vi "Test WebSocket Upgrade.vi"() -> ()   [LabVIEW 2020]
uses:
  HTTP Server/Trace Log.ctl
  HTTP Server/Trace Item.ctl
  HTTP Server/Processing Step.ctl
  <vilib>/IlluminatedG/IG HTTP Utils/HTTP Utils/Method.ctl
  Test WebSocket Page Controller/Test WebSocket Page Controller.lvclass
  C:/dev/illuminated-g/lv-http-server/HTTP Server/Handler/Handler.lvclass
  <vilib>/IlluminatedG/lv-msg-simple/Stream-Simple-Msg/Format.ctl
  <vilib>/IlluminatedG/lv-stream/stream/Stream.lvclass/Stream.ctl
  ddb143f1-6f1e-4d94-bb27-81deb445b84a.vi
  ddb143f1-6f1e-4d94-bb27-81deb445b84a.vi/2114ae84-1210-427f-82ef-c9e9e7f82752.vi
  <vilib>/IlluminatedG/lv-msg-simple/Stream-Simple-Msg/Endpoint/Write Flattened Data.vi
  ddb143f1-6f1e-4d94-bb27-81deb445b84a.vi/2114ae84-1210-427f-82ef-c9e9e7f82752.vi/850aaa44-16cf-4b05-95d8-204edf60ad4b.vi
  <vilib>/IlluminatedG/lv-stream/stream/Write Data.vi
  ddb143f1-6f1e-4d94-bb27-81deb445b84a.vi/2114ae84-1210-427f-82ef-c9e9e7f82752.vi/850aaa44-16cf-4b05-95d8-204edf60ad4b.vi/c20c7362-1c17-4c7a-86c1-0a7c7649dad4.vi
  <vilib>/IlluminatedG/lv-stream/stream/Dispatch Sniffer Data.vi
  <vilib>/IlluminatedG/lv-stream/stream/Prepared.vi
  <vilib>/IlluminatedG/lv-stream/Endpoint/Cast Sniffer Callback.vi
  <vilib>/IlluminatedG/IG WebSocket Stream/Stream-Websocket/Websocket Server/Websocket Server.lvclass
  C:/Program Files (x86)/National Instruments/LabVIEW 2020/vi.lib/IlluminatedG/lv-stream/Endpoint/Endpoint.lvclass
  HTTP Server/Server/Add Connection Handler.vi
  HTTP Server/Server/Add Request Handler.vi
  HTTP Server/Server/Add Route Handler.vi
  HTTP Server/Server/Add Controller Handler.vi
  HTTP Server/Server/Add Controller.vi
  HTTP Server/Server/Add Response Handler.vi
  HTTP Server/Server/Add Complete Handler.vi
  HTTP Server/Server/Add Exception Handler.vi
  <vilib>/IlluminatedG/lv-msg-simple/Stream-Simple-Msg/Manager/Endpoints and Formats.vi
  <vilib>/IlluminatedG/lv-msg-simple/Stream-Simple-Msg/Endpoint/Get Format.vi
  <vilib>/IlluminatedG/lv-msg-simple/Stream-Simple-Msg/Endpoint/Get Stream.vi
  <vilib>/Utility/error.llb/Error Cluster From Error Code.vi
  HTTP Server/Connection Handler/Connection Handler.lvclass
  HTTP Server/Request Handler/Request Handler.lvclass
  HTTP Server/Route Handler/Route Handler.lvclass
  HTTP Server/Controller Handler/Controller Handler.lvclass
  HTTP Server/Controller/Controller.lvclass
  HTTP Server/Response Handler/Response Handler.lvclass
  HTTP Server/Complete Handler/Complete Handler.lvclass
  HTTP Server/Exception Handler/Exception Handler.lvclass
  <vilib>/IlluminatedG/lv-msg-simple/Stream-Simple-Msg/Manager/Manager.lvclass
  HTTP Server/Server/Server.lvclass
  HTTP Server/Handler/Handler.lvclass
  <vilib>/IlluminatedG/lv-stream/stream/Stream.lvclass
  HTTP Server/RequestTraceLog/RequestTraceLog.lvclass
  <vilib>/ptbypt/NI_PtbyPt.lvlib
  <vilib>/IlluminatedG/lv-msg-simple/Stream-Simple-Msg/Stream-Simple-Msg.lvlib
  WebSocket Test UI Refs/WebSocket Test UI Refs.lvclass
  HTTP Server/HTTP Server.lvlib
  <vilib>/IlluminatedG/IG HTTP Utils/HTTP Utils/HTTP Utils.lvlib
panel:
  out "Last Greeting":string
  out ">0 Clients?":bool
  out "Sine Value":dbl format="%0.2f"
  in  "Refresh Traces":bool
  out "Traces":T1[](array[typedef]) {"Sending" format="%_6f"; "Expires" format="%<%X %x>T"; "Created" format="%<%X %x>T"; "Waiting" format="%_6f"; "Parsing" format="%_6f"; "Processing" format="%_6f"; "Items"."Time" format="%.6f"; "Items"."Duration" format="%.6f"}
  # "Request"
  # "Response"
  # "Session"
  # "Auth"
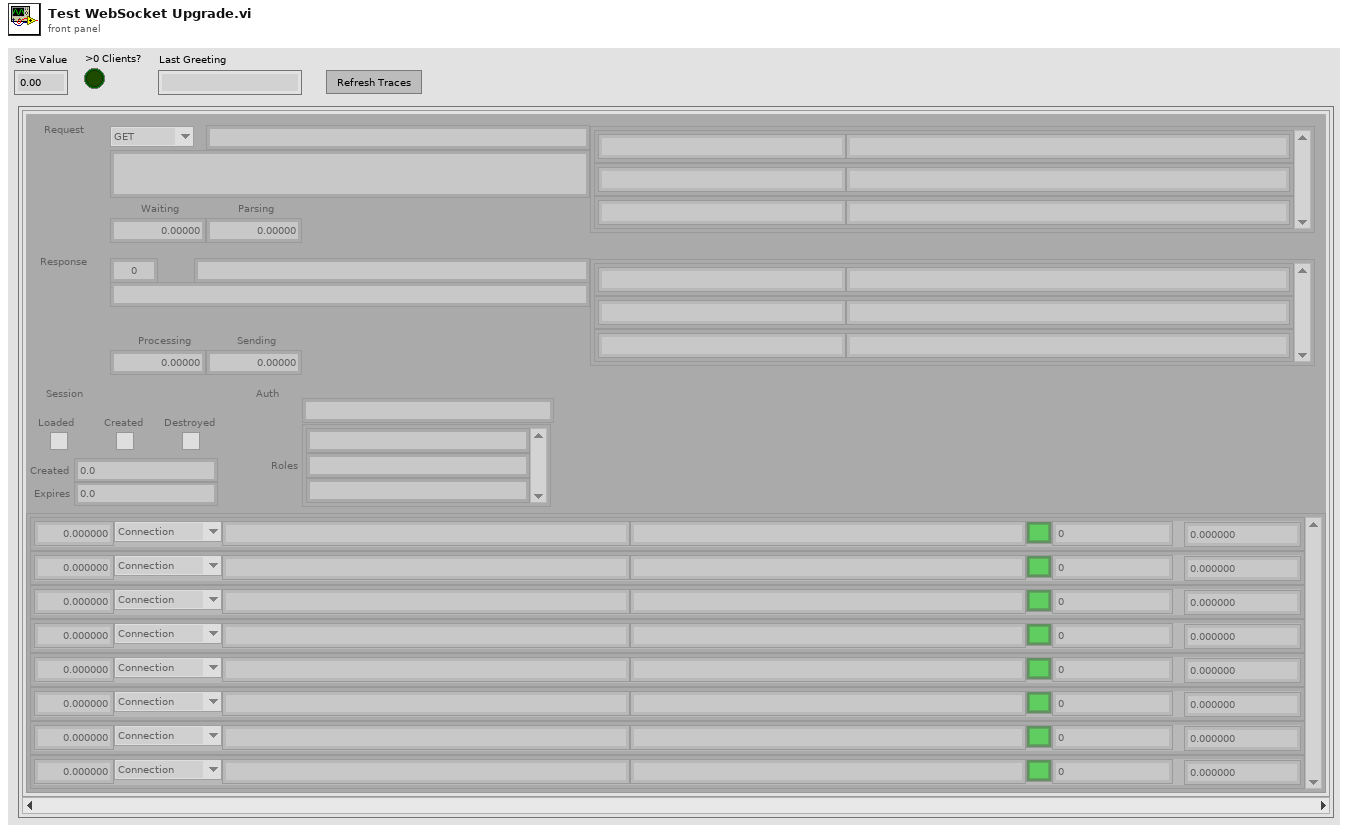
[diagram p1: front panel]
types:
  T1 = typedef "HTTP Server.lvlib/Trace Log.ctl" = cluster{"Items":T2[], "Client":string, "Target":string, "Response Type":string, "Processing":dbl, "Status":u16, "Method":T4, "Content Type":string, "Request Headers":cluster{"Name":string, "Value":string}[], "Parsing":dbl, "Waiting":dbl, "Identity":string, "Loaded":bool, "Created":bool, "Destroyed":bool, "Response Headers":cluster{"Name":string, "Value":string}[], "Created":dbl, "Expires":dbl, "Roles":string[], "Sending":dbl}
  T2 = typedef "HTTP Server.lvlib/Trace Item.ctl" = cluster{"Duration":dbl, "Step":T3, "Class":string, "Info":string, "Status":bool, "Code":i32, "Time":dbl}
  T3 = typedef "HTTP Server.lvlib/Processing Step.ctl" = enum16{"Connection", "Request", "Routing", "Controller Init", "Controller", "Response", "Complete", "Exception"}
  T4 = typedef "HTTP Utils.lvlib/Method.ctl" = enum16{"GET", "HEAD", "POST", "PUT", "DELETE", "CONNECT", "OPTIONS", "TRACE", "PATCH"}
  T5 = typedef "Stream-Simple-Msg.lvlib/Format.ctl" = enum16{"LabVIEW Binary", "JSON"}
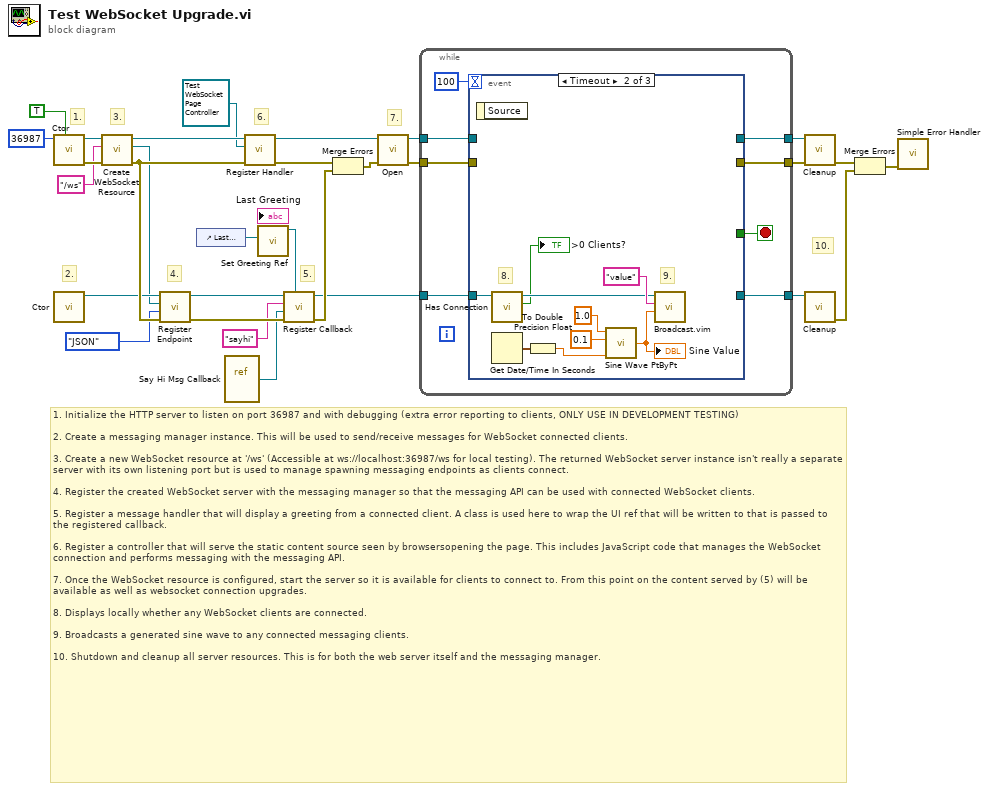
[diagram p0: block diagram]
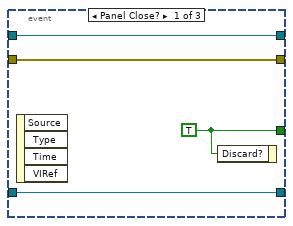
[diagram p2: hidden frame]
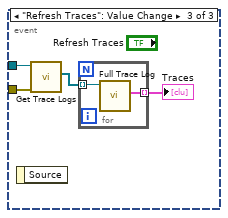
[diagram p3: hidden frame]
diagram:
  # "10."
  # "7."
  # "5."
  # "1. Initialize the HTTP server to listen on port 36987 and with debugging (extra error reporting to clients, ONLY USE IN DEVELOPMENT TESTING)\n\n2. Create a messaging manager instance. This will be used to send/receive messages for WebSocket connected clients.\n\n3. Create a new WebSocket resource at '/ws' (Accessible at ws://localhost:36987/ws for local testing). The returned WebSocket server instance isn't really a separate server with its own listening port but is used to manage spawning messaging endpoints as clients connect.\n\n4. Register the created WebSocket server with the messaging manager so that the messaging API can be used with connected WebSocket clients.\n\n5. Register a message handler that will display a greeting from a connected client. A class is used here to wrap the UI ref that will be written to that is passed to the registered callback.\n\n6. Register a controller that will serve the static content source seen by browsersopening the page. This includes JavaScript code that manages the WebSocket connection and performs messaging with the messaging API.\n\n7. Once the WebSocket resource is configured, start the server so it is available for clients to connect to. From this point on the content served by (5) will be available as well as websocket connection upgrades.\n\n8. Displays locally whether any WebSocket clients are connected.\n\n9. Broadcasts a generated sine wave to any connected messaging clients.\n\n10. Shutdown and cleanup all server resources. This is for both the web server itself and the messaging manager."
  # "6."
  # "4."
  # "3."
  # "2."
  # "1."
  n1 = call <vilib>:"Ctor.vi"("Debug (F)"=TRUE, "HTTP Port (80)"=u16 36987 ("Port (8080)")) -> ("error out"=w24:errorcluster, "Server out"=w25:refnum<class "Server.lvclass">)  [unwired: 8 in]
  n2 = call <vilib>:"Ctor.vi"() -> ("Manager out"=w14:refnum<class "Manager.lvclass">)  [unwired: 10 in, 1 out]
  n3 = call "Create WebSocket Resource.vi"("error in (no error)"=w24, "Path"="/ws", "Server in"=w25) -> ("error out"=w28:errorcluster, "WS Server"=w10:refnum<class "Websocket Server.lvclass">, "Server out"=w17:refnum<class "Server.lvclass">)  [unwired: 6 in]
  n4 = call <vilib>:"Register Endpoint.vi"("error in (no error)"=w28, "Format (LabVIEW Binary)"=Format."JSON", "Stream:Endpoint"=w10, "Manager in"=w14) -> ("error out"=w30:errorcluster, "Manager out"=w8:refnum<class "Manager.lvclass">)  [unwired: 6 in]
  n5 = control-ref of="Last Greeting"() -> (w4:refnum<vi>)
  n6 = vi-ref "Say Hi Msg Callback.vi"() -> (w5:refnum<vi>)
  n7 = call "Register Handler.vi"("error in (no error)"=w28, "Handler"=refnum<class "Test WebSocket Page Controller.lvclass"> refnum ("Test WebSocket Page Controller.lvclass"), "Server in"=w17) -> ("error out"=w12:errorcluster, "Server out"=w16:refnum<class "Server.lvclass">)  [unwired: 7 in]
  n8 = call "Set Greeting Ref.vi"("Last Greeting"=w4) -> ("WebSocket Test UI Refs out"=w3:refnum<class "WebSocket Test UI Refs.lvclass">)  [unwired: 9 in, 1 out]
  n9 = call <vilib>:"Register Callback.vi"("Owner"=w3, "error in (no error)"=w30, "Callback"=w5, "Message ID"="sayhi", "Manager in"=w8) -> ("error out"=w29:errorcluster, "Manager out"=w6:refnum<class "Manager.lvclass">)  [unwired: 5 in]
  n10 = Merge Errors(w12, w29) -> (w9:errorcluster)
  n11 = call "Open.vi"("error in (no error)"=w9, "Server in"=w16) -> ("error out"=w18:errorcluster, "Server out"=w19:refnum<class "Server.lvclass">)  [unwired: 8 in]
  n12 = while {
    tunnel: w19 -> [w38]
    tunnel: w18 -> [w37]
    tunnel: [w35] -> w22
    tunnel: [w34] -> w21
    tunnel: w6 -> [w32]
    tunnel: [w31] -> w11
    stop <- w36 stop-if-true
    n13 = event shown="[1] Timeout" {
      selector: _ -> [_ _ _]
      dyn-events: _ -> [_ _ _]
      timeout: 100 -> [_ _ _]
      tunnel: w38 -> [w42 _ w55]
      tunnel: w37 -> [w41 _ w54]
      tunnel: [w39 _ _] -> w36
      tunnel: [w42 _ _] -> w35
      tunnel: [w41 _ _] -> w34
      tunnel: w32 -> [w40 w47 _]
      tunnel: [w40 _ _] -> w31
      event Panel Close? {
        w39 = TRUE
        n14 = event-data() -> ()  [unwired: 1 in, 4 out]
        n15 = event-data("Discard?"=w39) -> ()  [unwired: 1 in, 1 out]
      }
      event Timeout {
        # "9."
        # "8."
        n16 = event-data() -> ()  [unwired: 1 in, 1 out]
        n17 = call <vilib>:"Has Connection.vi"("Manager in"=w47) -> ("Connected"=→">0 Clients?":bool, "Manager out"=w46:refnum<class "Manager.lvclass">)  [unwired: 8 in, 1 out]
        n18 = Get Date/Time In Seconds() -> (seconds since 1Jan1904=w44:timestamp)
        n19 = To Double Precision Float(number=w44) -> (double precision float=w43:dbl)
        n20 = call <vilib>:"Sine Wave PtByPt.vi"("time"=w43, "frequency"=0.1, "amplitude"=1.0) -> ("sine wave"=w48:dbl)  [unwired: 1 in]
        "Sine Value" <- w48
        n21 = call "Broadcast.vim"("Data"=w48, "ID"="value", "Manager in"=w46) -> ()  [unwired: 7 in, 2 out]
      }
      event "Refresh Traces": Value Change {
        n22 = event-data() -> ()  [unwired: 1 in, 1 out]
        n23 = call "Get Trace Logs.vi"("error in (no error)"=w54, "Server in"=w55) -> ("Trace Logs"=w53:refnum<class "RequestTraceLog.lvclass">[])  [unwired: 7 in, 2 out]
        n24 = for {
          tunnel: w53 -> [w57] mode=indexing
          tunnel: [w56] -> w52 mode=indexing
          n25 = call "Full Trace Log.vi"("RequestTraceLog in"=w57) -> ("Trace Log"=w56:T1)  [unwired: 8 in, 2 out]
        }
        "Traces" <- w52
      }
    }
  }
  n26 = call <vilib>:"Cleanup.vi"("error in (no error)"=w21, "Server in"=w22) -> ("error out"=w20:errorcluster)  [unwired: 9 in]
  n27 = call <vilib>:"Cleanup.vi"("Manager in"=w11) -> ("error out"=w1:errorcluster)  [unwired: 10 in]
  n28 = Merge Errors(w20, w1) -> (w2:errorcluster)
  n29 = call <vilib>:"Simple Error Handler.vi"("error in (no error)"=w2) -> ()  [unwired: 4 in, 5 out]
